vi "PXI_Host_Bool_Write_OldMethod_Benchmark.vi"() -> ()   [LabVIEW 2018]
uses:
  <vilib>/Platform/TimedLoop/XDataNode/timing_clust.ctl
  <vilib>/Platform/TimedLoop/XDataNode/nitl_modes.ctl
  <vilib>/Platform/TimedLoop/XDataNode/wakeup.ctl
  <vilib>/NI/LVFPGA Adv Session Resources/OpenByNameSubVI.vi
  <vilib>/rvi/interface/common/dynamic/niFpgaEscapeDelimiterAndNull.vi
  <vilib>/Utility/error.llb/Error Cluster From Error Code.vi
  <vilib>/rvi/errors/niLvFpgaAdjustHostInterfaceError.vi
  <vilib>/FPGAPlugInAG/Dynamic/niLvFpga_Close_Dynamic.vi
  <vilib>/platform/TimedLoop/XDataNode/XDataNode.xnode
  <vilib>/NI/LVFPGA Adv Session Resources/OpenByName.xnode
  <vilib>/rvi/interface/nirviReadWriteControl/nirviReadWriteControl.xnode
  <vilib>/rvi/interface/nirviCloseFPGA/nirviCloseFPGA.xnode
  NiFpgaLv.dll
  <vilib>/rvi/interface/Simulation/niFpgaSimulationCallBeginRW.vi
  cRIO RT/FPGA Bitfile Register Operations/Scalar IO Operations/FPGA Register IO.lvlib
  <vilib>/Platform/TimedLoop/XDataNode/XDNodeRunTimeDep.lvlib
  <vilib>/NI/LVFPGA Adv Session Resources/LVFPGAAdvSessionResources.lvlib
panel:
  out "Maximum(s)":dbl
  out "Standard deviation":dbl
  out "Waveform Graph":dbl[](graph)
  out "error out 2":errorcluster
  out "Execution time (s)":dbl
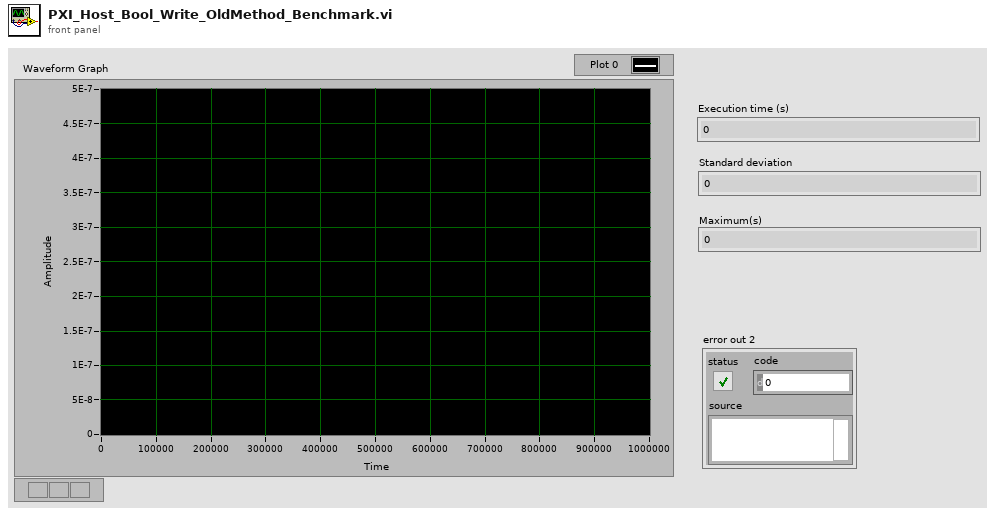
[diagram p1: front panel]
types:
  T1 = typedef "XDNodeRunTimeDep.lvlib/timing_clust.ctl" = cluster{"Expected End [f-1]":u64, "Actual End [f-1]":u64, "Finished Late? [f-1]":bool, "Expected End [i-1]":u64, "Actual End [i-1]":u64, "Finished Late? [i-1]":bool, "Expected Start [i]":u64, "Actual Start [i]":u64, "Expected Start [f]":u64, "Actual Start [f]":u64, "Source Name":string, "Structure Name":string, "Period":i64, "Deadline":i64, "Offset":i64, "Start":i64, "Priority":i32, "Timeout":i32, "Mode":T2, "Wakeup Reason":T3, "Error":errorcluster, "Source Type":string, "Secondary Source Type":string, "Global End Time":u64, "Global Start Time":u64, "Frame Duration":u64, "Iteration Duration":u64, "Assigned CPU":i32, "I/O Scan Engine Mode":u32}
  T2 = typedef "XDNodeRunTimeDep.lvlib/nitl_modes.ctl" = enum32{"No Change", "Process missed periods, maintain original phase", "Discard missed periods, maintain original phase", "Process missed periods, ignore original phase", "Discard missed periods, ignore original phase"}
  T3 = typedef "XDNodeRunTimeDep.lvlib/wakeup.ctl" = enum32{"Normal", "Aborted", "Asynchronous wakeup", "Timing source error", "Timed loop error", "Timeout"}
  T4 = cluster{"Name":string, "Depth":u32, "Write? (Deprecated:Use Implementation)":bool, "Physical Channel":u32, "Base Address":u32, "Data Width":u32, "Data Type":enum32{"Boolean", "I8", "I16", "I32", "I64", "U8", "U16", "U32", "U64", "FXP", "CustomControl", "SGL"}, "FXP Properties":variant, "Write Window Address":u32, "Implementation":enum16{"niFpgaTargetToHost", "niFpgaHostToTarget", "niFpgaPeerToPeerWriter", "niFpgaPeerToPeerReader", "niCoreTargetToHost", "niCoreHostToTarget"}, "Control Set":u32}[]
  T5 = cluster{"Name":string, "type":variant, "indicator?":bool}[]
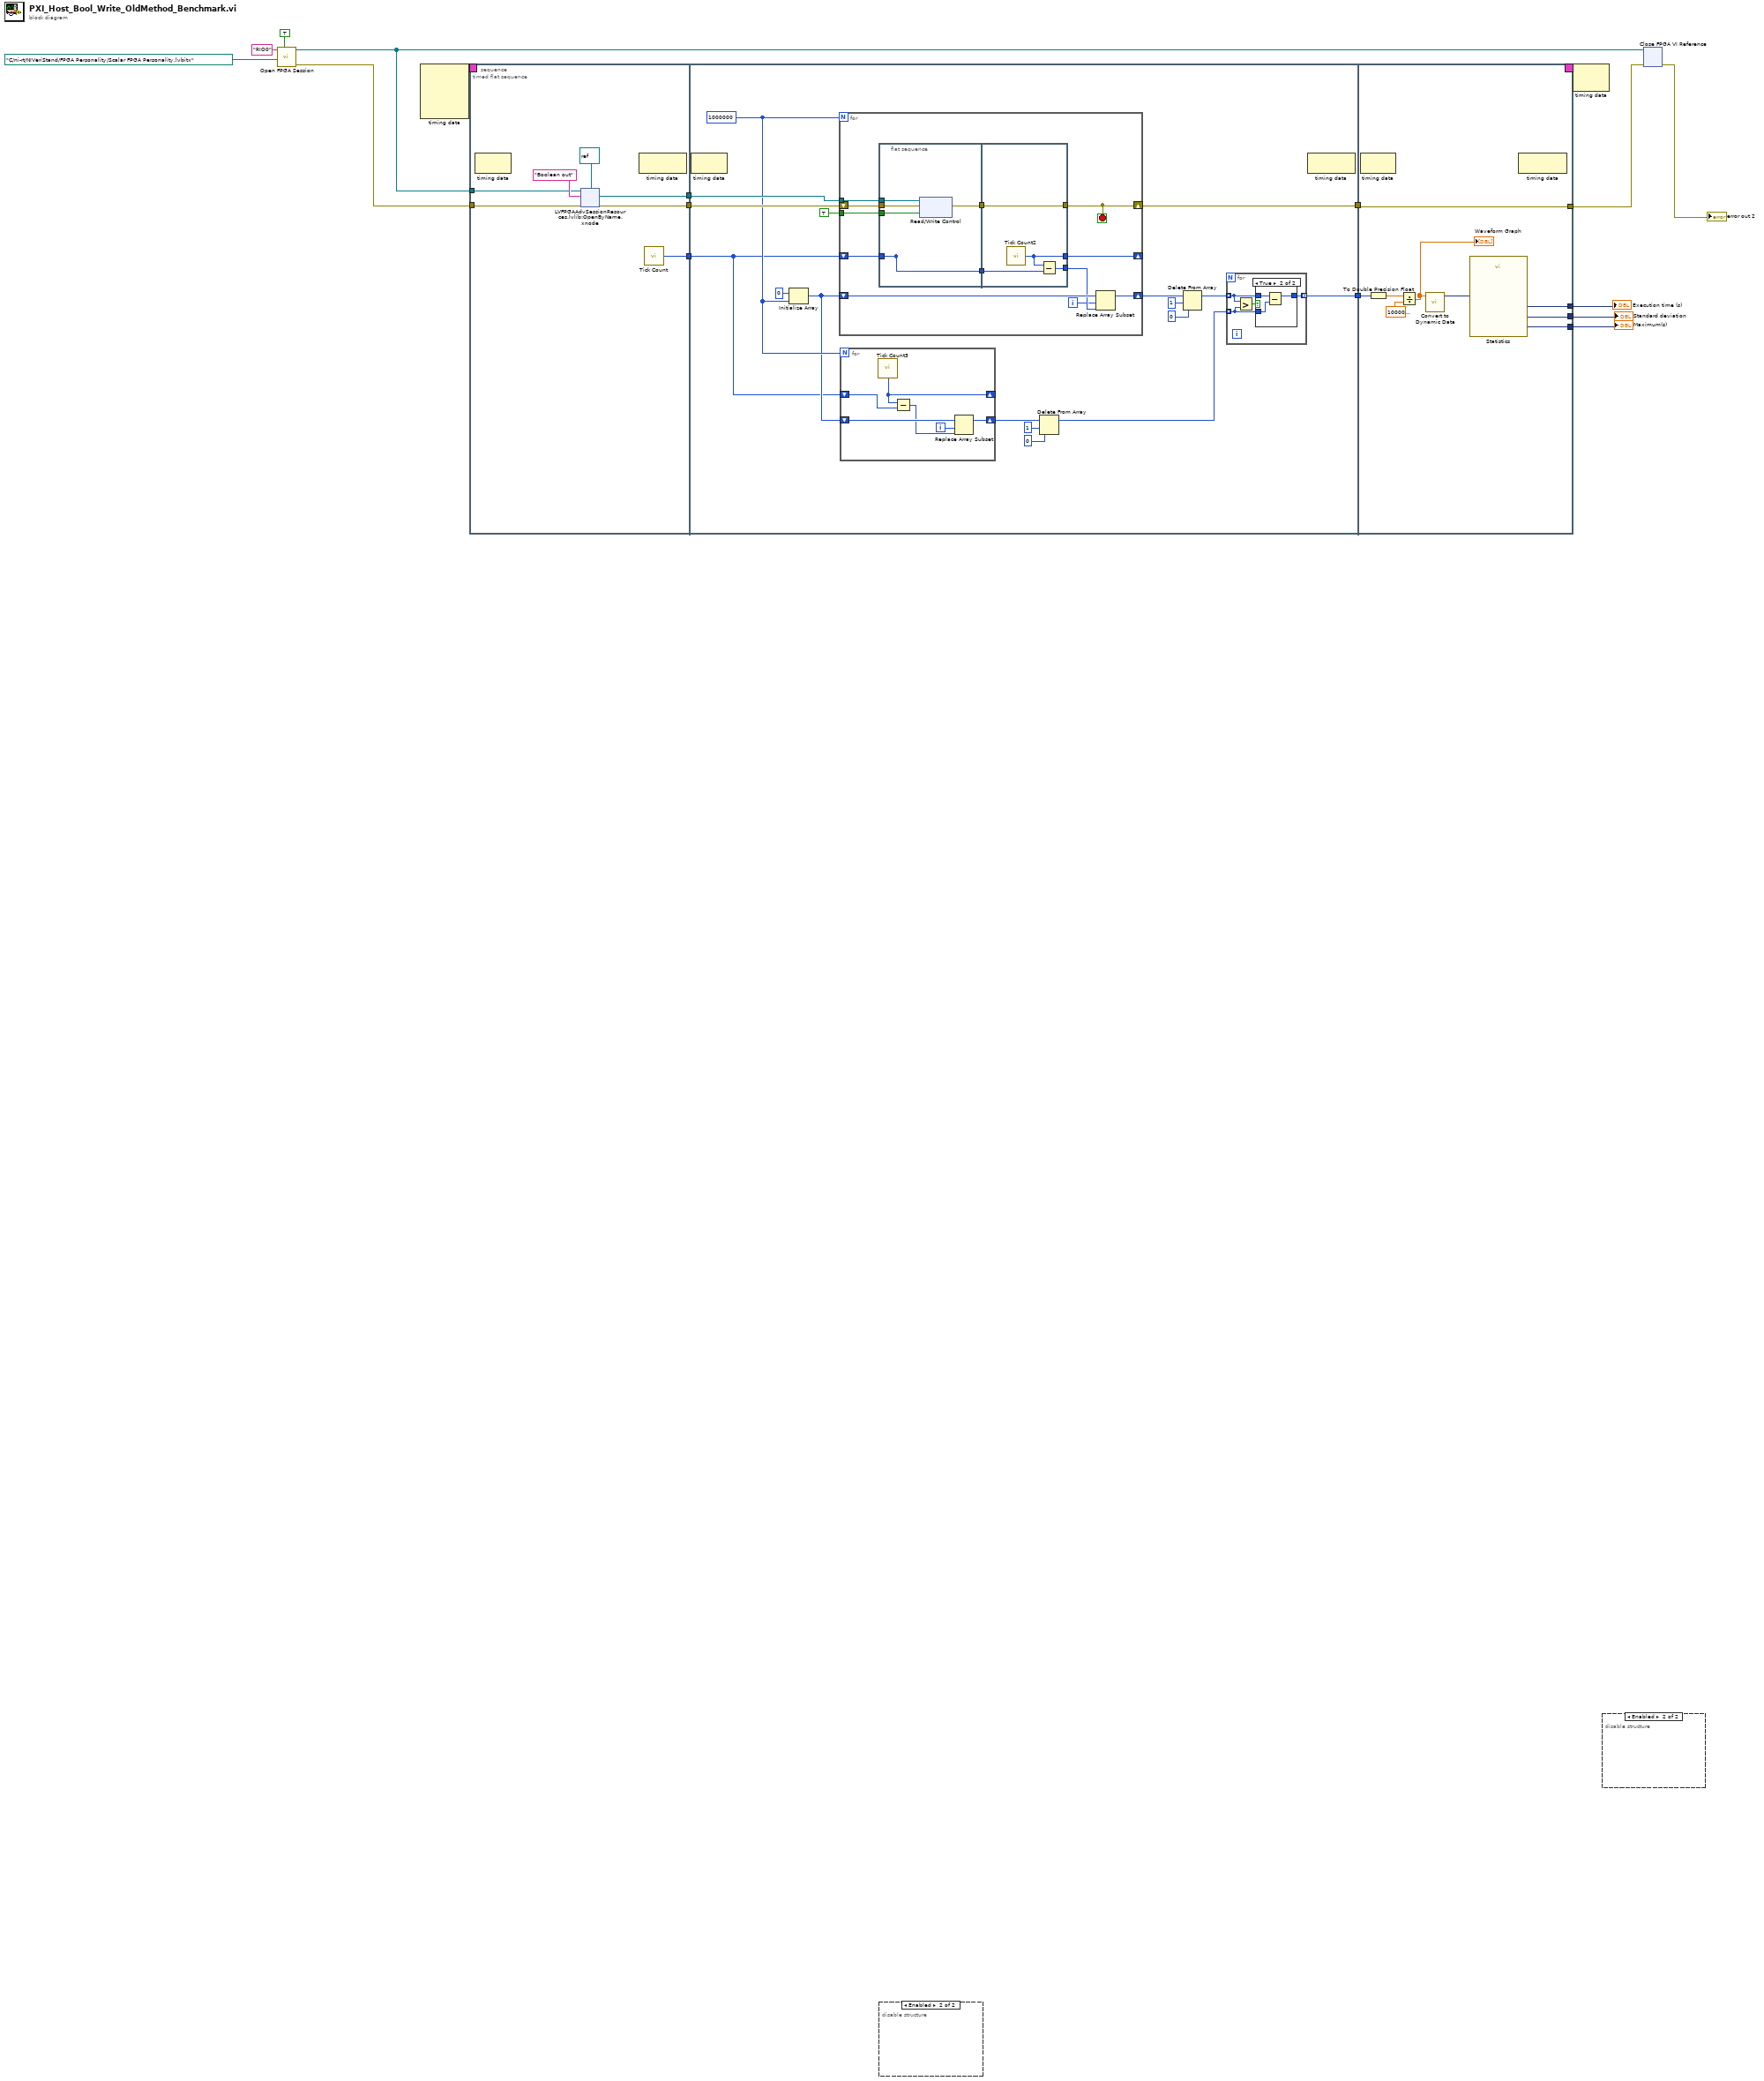
[diagram p0: block diagram]
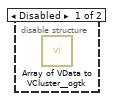
[diagram p3: hidden frame]
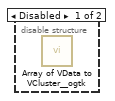
[diagram p4: hidden frame]
diagram:
  n1 = call "Open FPGA Session.vi"("run when loaded (T)"=TRUE, "bitfile path"=path "C:/ni-rt/NIVeriStand/FPGA Personality/Scalar FPGA Personality.lvbitx", "device address"="RIO0") -> ("error out"=w7:errorcluster, "bitfile reference out"=w1:refnum<k20>)  [unwired: 6 in, 1 out]
  n2 = node-c288() -> (w12:T1)  [unwired: 4 in]
  n3 = timed-sequence {
    timing: w12 -> [_]
    timing-out: [_] -> w11
    tunnel: w7 -> [w15]
    tunnel: [w20] -> w6
    tunnel: [w18] -> w4
    tunnel: [w17] -> w3
    tunnel: [w16] -> w2
    tunnel: w1 -> [w14]
    n4 = timed-flat-sequence {
      tunnel: [w25] -> w23
      tunnel: [w24] -> w22
      tunnel: [w30] -> w19
      tunnel: w15 -> [w27]
      tunnel: w14 -> [w26]
      tunnel: w23 -> [w62]
      tunnel: [w61] -> w21
      tunnel: w22 -> [w60]
      tunnel: w19 -> [w49]
      tunnel: [w47] -> w13
      tunnel: w21 -> [w108]
      tunnel: [w108] -> w20
      tunnel: [w106] -> w18
      tunnel: [w103] -> w17
      tunnel: [w102] -> w16
      tunnel: w13 -> [w101]
      frame #0 {
        n5 = node-c288() -> ()  [unwired: 1 in, 1 out]
        n6 = xnode "LVFPGAAdvSessionResources.lvlib:OpenByName.xnode"("FPGA VI Reference in"=w26, "Resource name in"="Boolean out", "Single resource reference type in"=refnum<k20> refnum ("Type"), "Error in"=w27) -> ("Single resource reference out"=w24:refnum<k20>, "Error out"=w25:errorcluster)  [unwired: 1 out]
        n7 = node-c288() -> ()  [unwired: 1 in, 1 out]
        n8 = call "Tick Count"() -> ("Tick Count(Ticks)"=w30:u32)
      }
      frame #1 {
        w51 = 1000000
        n9 = node-c288() -> ()  [unwired: 1 in, 1 out]
        n10 = Initialize Array(u32 0, w51) -> (w50:u32[])
        n11 = for {
          N: w51 -> [_]
          tunnel: w60 -> [w89]
          shift-right: [w87] -> _
          shift-left: w49 -> [w86]
          shift-right: [w82] -> w58
          shift-left: w50 -> [w84]
          shift-right: [w80] -> w61
          shift-left: w62 -> [w90]
          tunnel: TRUE ("Value") -> [w79]
          i -> [w81]
          stop <- w80 stop-if-true
          n12 = flat-sequence {
            tunnel: w90 -> [w94]
            tunnel: w89 -> [w92]
            tunnel: [w93] -> w88
            tunnel: [w95] -> _
            tunnel: w86 -> [w95]
            tunnel: [w95] -> w85
            tunnel: w79 -> [w91]
            tunnel: [w99] -> w80
            tunnel: w88 -> [w99]
            tunnel: [w98] -> w87
            tunnel: w85 -> [w97]
            tunnel: [w96] -> w83
            frame #0 {
              n13 = xnode "Read/Write Control"("FPGA VI Reference In"=w92, "error in"=w94, "Value"=w91) -> ("error out"=w93:errorcluster)  [unwired: 1 out]
            }
            frame #1 {
              n14 = call "Tick Count2"() -> ("Tick Count(Ticks)"=w98:u32)
              n15 = Subtract(x=w98, y=w97) -> (x-y=w96:u32)
            }
          }
          n16 = Replace Array Subset(array=w84, new element=w83, index=w81) -> (w82:u32[])
        }
        n17 = for {
          N: w51 -> [_]
          shift-right: [w71] -> w52
          shift-left: w50 -> [w74]
          shift-right: [w76] -> _
          shift-left: w49 -> [w75]
          i -> [w72]
          n18 = call "Tick Count3"() -> ("Tick Count(Ticks)"=w76:u32)
          n19 = Subtract(x=w76, y=w75) -> (x-y=w73:u32)
          n20 = Replace Array Subset(array=w74, new element=w73, index=w72) -> (w71:u32[])
        }
        n21 = Delete From Array(array=w52, length=1, index=0) -> (array with subset deleted=w46:u32[])  [unwired: 1 out]
        n22 = Delete From Array(array=w58, length=1, index=0) -> (array with subset deleted=w48:u32[])  [unwired: 1 out]
        n23 = for {
          tunnel: [w66] -> w47 mode=indexing
          tunnel: w48 -> [w65] mode=indexing
          tunnel: w46 -> [w64] mode=indexing
          n24 = Greater?(x=w65, y=w64) -> (0:w63:bool)
          n25 = case shown="True" w63 {
            tunnel: w65 -> [w67 w70]
            tunnel: w64 -> [_ w69]
            tunnel: [w67 w68] -> w66
            frame False {
            }
            frame True {
              n26 = Subtract(x=w70, y=w69) -> (x-y=w68:u32)
            }
          }
        }
        n27 = node-c288() -> ()  [unwired: 1 in, 1 out]
      }
      frame #2 {
        n28 = node-c288() -> ()  [unwired: 1 in, 1 out]
        n29 = To Double Precision Float(number=w101) -> (double precision float=w105:dbl[])
        n30 = Divide(x=w105, y=1000000000.0) -> (x/y=w100:dbl[])
        "Waveform Graph" <- w100
        n31 = call "Convert to Dynamic Data"("Array"=w100) -> ("Dynamic Data Type"=w107:dynamicdata)  [unwired: 3 in]
        n32 = call "Statistics"("Signals"=w107) -> ("Standard Dev"=w103:dynamicdata, "Arithmetic Mean"=w106:dynamicdata, "Maximum"=w102:dynamicdata)  [unwired: 23 in, 1 out]
        n33 = node-c288() -> ()  [unwired: 1 in, 1 out]
      }
    }
  }
  "Execution time (s)" <- w4
  "Standard deviation" <- w3
  "Maximum(s)" <- w2
  n34 = disable-structure shown="Enabled" {
    frame Disabled {
      n35 = call <userlib>:"Array of VData to VCluster__ogtk.vi"() -> ()  [unwired: 10 in, 2 out]
    }
    frame Enabled {
    }
  }
  n36 = node-c288(w11) -> ()  [unwired: 1 out]
  n37 = disable-structure shown="Enabled" {
    frame Disabled {
      n38 = call <userlib>:"Array of VData to VCluster__ogtk.vi"() -> ()  [unwired: 10 in, 2 out]
    }
    frame Enabled {
    }
  }
  n39 = xnode "Close FPGA VI Reference"("FPGA VI Reference In"=w1, "error in"=w6) -> ("error out"=→"error out 2":errorcluster)
